vi "getRandomColor.vi"(8 "error in (no error)":errorcluster, 11 "Flightweight Pattern Demo in":refnum<class "Flightweight Pattern Demo.lvclass">) -> (0 "error out":errorcluster, 2 "Color":string, 3 "Flightweight Pattern Demo out":refnum<class "Flightweight Pattern Demo.lvclass">)   [LabVIEW 2017, in "Flightweight Pattern Demo.lvclass"]
uses:
  Flightweight Pattern Demo.lvclass
  Flightweight Pattern Demo.lvclass/Flightweight Pattern Demo.ctl
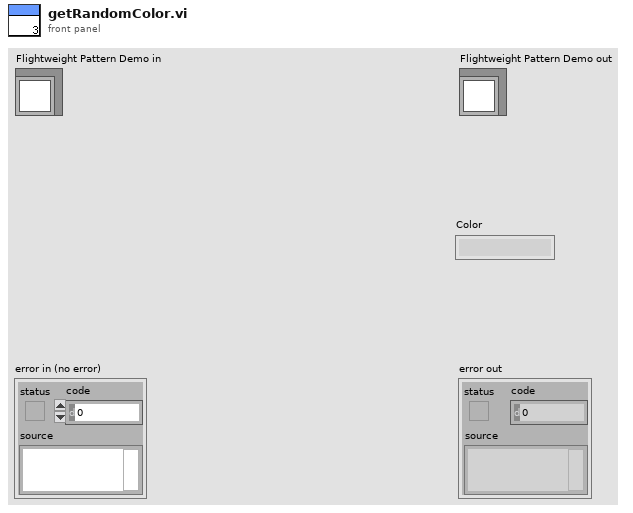
[diagram p1: front panel]
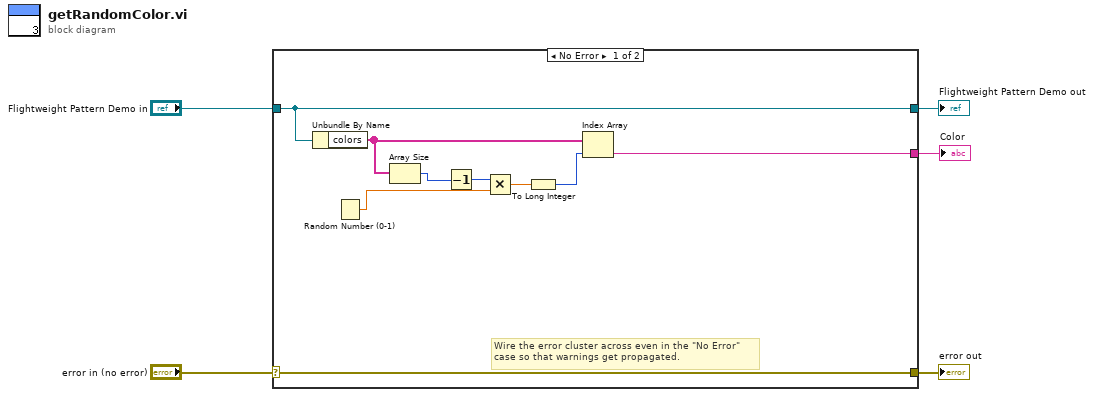
[diagram p0: block diagram]
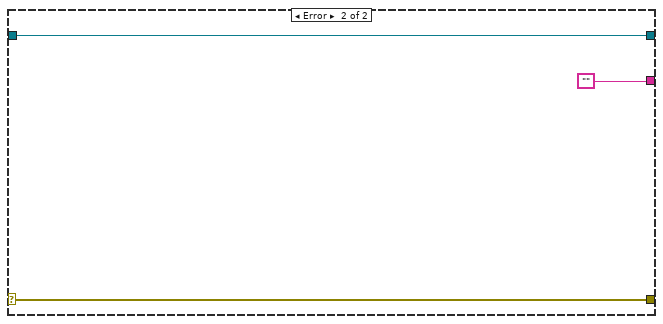
[diagram p2: hidden frame]
diagram:
  n1 = case shown="No Error" "error in (no error)" {
    selector: "error in (no error)" -> [w14 w17]
    tunnel: [w14 w17] -> w4
    tunnel: [w13 w16] -> w2
    tunnel: "Flightweight Pattern Demo in" -> [w13 w16]
    tunnel: [w9 ""] -> w1
    frame No Error {
      # "Wire the error cluster across even in the \"No Error\"\ncase so that warnings get propagated."
      n2 = Unbundle By Name(w13) -> ("colors"=w10:string[])
      n3 = Random Number (0-1)() -> (number: 0 to 1=w11:dbl)
      n4 = Array Size(array=w10) -> (size(s)=w12:i32)
      n5 = Decrement(x=w12) -> (x-1=w6:i32)
      n6 = Multiply(x=w6, y=w11) -> (x*y=w7:dbl)
      n7 = To Long Integer(number=w7) -> (32bit integer=w8:i32)
      n8 = Index Array(array=w10, index=w8) -> (element=w9:string)
    }
    frame Error {
    }
  }
  "error out" <- w4
  "Flightweight Pattern Demo out" <- w2
  "Color" <- w1
